vi "QVA_DeleteAllVariantAttributes.vi"(0 "QueueIn":refnum<queue>, 5 "ErrorIn":errorcluster, 9 "Timeout":i32=-1) -> (14 "QueueOut":refnum<queue>, 16 "Timeout":bool, 19 "ErrorOut":errorcluster)   [LabVIEW 2016]
doc: "Löscht alle Variant Attributes aus dem QVA\n\nsige / 3.12.13"
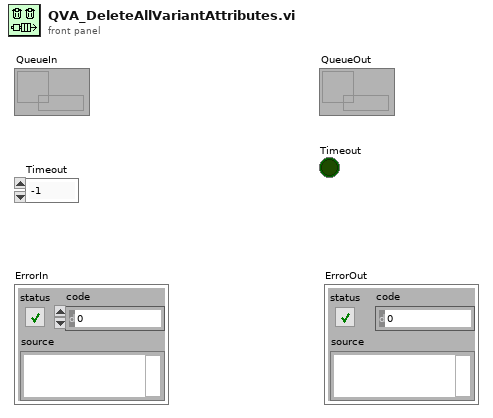
[diagram p1: front panel]
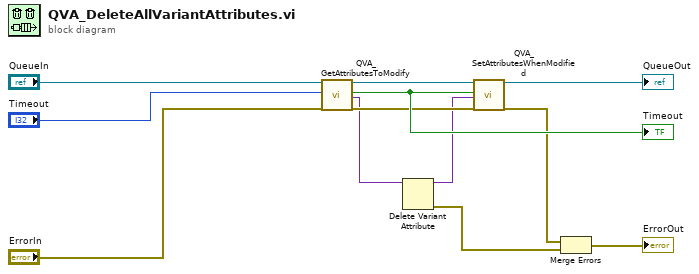
[diagram p0: block diagram]
diagram:
  n1 = call "QVA_GetAttributesToModify.vi"("QueueIn"="QueueIn", "Timeout"="Timeout", "ErrorIn"="ErrorIn") -> ("QueueOut"=w6:refnum<queue>, "Timeout"=w9:bool, "VariantData"=w3:variant, "ErrorOut"=w4:errorcluster)  [unwired: 13 in]
  "Timeout" <- w9
  n2 = Delete Variant Attribute(7:w3) -> (0:w1:errorcluster, 3:w2:variant)  [unwired: 2 in, 1 out]
  n3 = call "QVA_SetAttributesWhenModified.vi"("QueueIn"=w6, "SkipAfterTimeout"=w9, "VariantData"=w2, "ErrorIn"=w4) -> ("QueueOut"=→"QueueOut":refnum<queue>, "ErrorOut"=w5:errorcluster)  [unwired: 14 in]
  n4 = Merge Errors(w5, w1) -> (→"ErrorOut":errorcluster)
